vi "Core Actor - Close User Events.vi"(8 "error in (no error)":errorcluster, 11 "Child_2_Class in":refnum<class "Console_Class.lvclass">) -> (0 "error out":errorcluster, 3 "Child_2_Class out":refnum<class "Console_Class.lvclass">)   [LabVIEW 2023, in "Console_Actor.lvlib" / "Console_Class.lvclass"]
uses:
  Console_Class.lvclass
  Usr Ev/Child_2 - Ctrl - Action.ctl
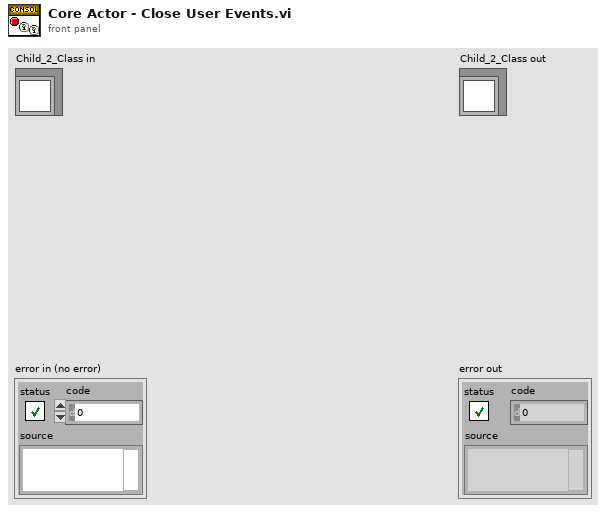
[diagram p1: front panel]
types:
  T1 = typedef "Console_Actor.lvlib/Console_Class.lvclass/Child_2 - Ctrl - Action.ctl" = enum16{"Reg Ev", "Get Refs", "Close Ev", "Populate Enum with Events"}
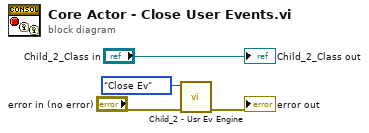
[diagram p0: block diagram]
diagram:
  n1 = call "Child_2 - Usr Ev Engine.vi"("error in (no error)"="error in (no error)", "Action"=Child_2_-_Ctrl_-_Action."Close Ev") -> ("error out"=→"error out":errorcluster)  [unwired: 6 in, 3 out]
  "Child_2_Class out" <- "Child_2_Class in"
